vi "Refprop_Example_main_V10.vi"() -> ()   [LabVIEW 2016]
doc: "Sample vi to demonstrate the use of REFPROP in LabVIEW developed by Ken Pop Yan Ding.\nThare are also some VIs written by Greg Sussman in this example.Thanks Greg Sussman."
panel:
  out "INFO_OUT":T1
  out "1st run":bool
  out "name out":string
  out "o2":string
  out "o1":string
  out "error out":errorcluster caption="Error Out"
  out "refprop _main_directory":string
  out "DLL Version Number":dbl format="%.2g"
  in  "InpCode":T2(ring)=enum."TP"
  out "data":string[][](table)=[["0", "T", "40.917420"], ["1", "P", "632.917420"], ["2", "H", "466.332574"], ["3", "S", "2.054657"], ["4", "DV", "18.926081"], ["5", "DL", "18.926081"], ["6", "E", "432.891028"], ["7", "CV", "0.758226"], ["8", "CP", "0.924261"], ["9", "W", "194.299169"], ["10", "Q", "998.000000"]]
  in  "input_2":dbl=632.0
  in  "input_1":dbl=40.0
  in  "Units":enum16{"SI"}(ring)
  in  "Fluid Name":u16(ring)=17 items=["R401A.MIX", "R401B.MIX", "R401C.MIX", "R402A.MIX", "R402B.MIX", "R403A.MIX", "R403B.MIX", "R405A.MIX", "R406A.MIX", "R407A.MIX", "R407B.MIX", "R407C.MIX", "R407D.MIX", "R407E.MIX", "R408A.MIX", "R409A.MIX", "R409B.MIX", "R410A.MIX", "R410B.MIX", "R411A.MIX", "R411B.MIX", "R412A.MIX", "R413A.MIX", "R414B.MIX", "R500.MIX", "R501.MIX", "R502.MIX", "R503.MIX", "R504.MIX", "R507A.MIX", "R508A.MIX", "R508B.MIX", "R509A.MIX", "ammonia.fld", "butane.fld", "ethane.fld", "propane.fld", "R11.fld", "R113.fld", "R114.fld", "R115.fld", "R116.fld", "R12.fld", "R123.fld", "R124.fld", "R125.fld", "R13.fld", "R134a.fld", "R141b.fld", "R142b.fld", "R143a.fld", "R152a.fld", "R218.fld", "R22.fld", "R227ea.fld", "R23.fld", "R236ea.fld", "R236fa.fld", "R245ca.fld", "R245fa.fld", "R32.fld", "R41.fld", "RC318.fld", "water.fld"]
  # "-->"
  # "-->"
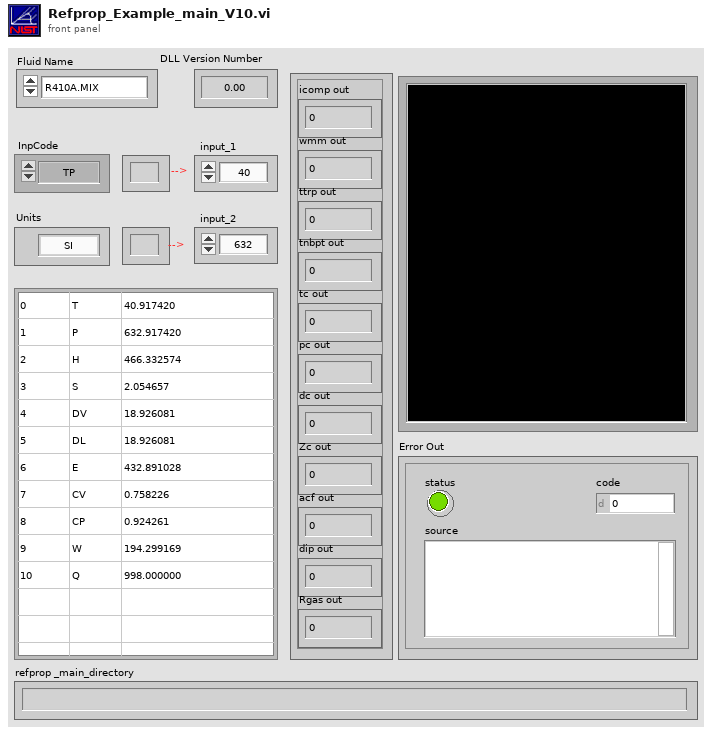
[diagram p1: front panel]
types:
  T1 = cluster{"icomp out":i32, "wmm out":dbl, "ttrp out":dbl, "tnbpt out":dbl, "tc out":dbl, "pc out":dbl, "dc out":dbl, "Zc out":dbl, "acf out":dbl, "dip out":dbl, "Rgas out":dbl}
  T2 = enum16{"0", "PS", "HS", "T", "P", "TP", "TH", "TS", "PH", "PQ", "TQ"}
  T3 = typedef "Mixture Composition cluster_d.ctl" = cluster{"Mixture Name":string, "Molecular weight (g/mol)":dbl, "Critical temperature (K)":dbl, "Critical Pressure (kPa)":dbl, "Critical Density (mol/L)":dbl, "# Components":i32, "Fluid File Paths":path[], "Component molar fractions":dbl[], "Refprop Main Directory":path, "DLL Version Number":dbl}
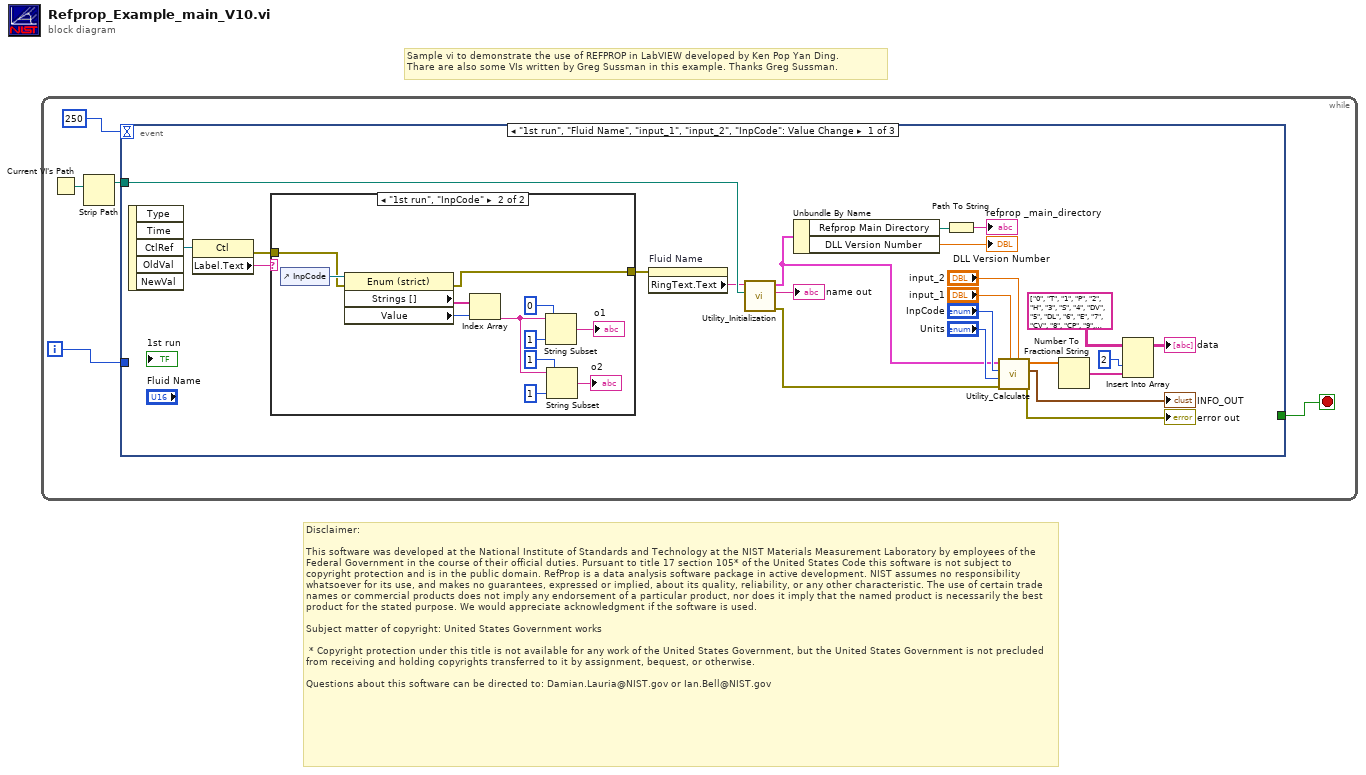
[diagram p0: block diagram]
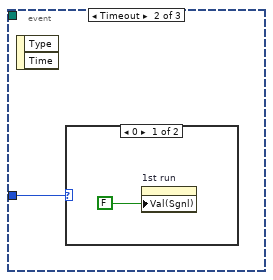
[diagram p3: hidden frame]
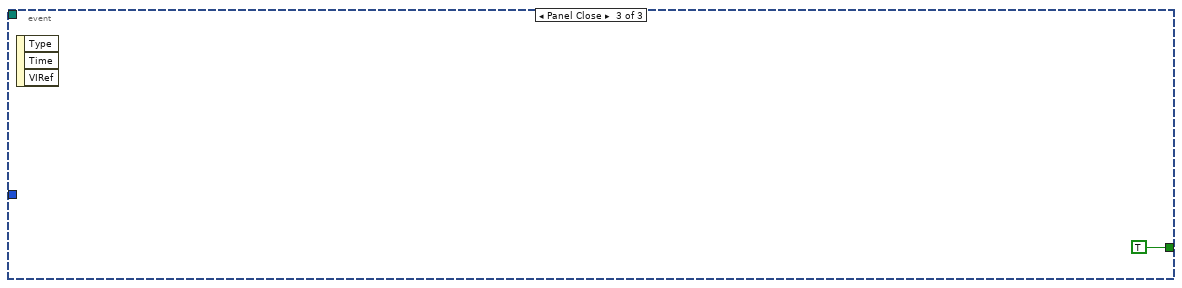
[diagram p5: hidden frame]
diagram:
  # "Sample vi to demonstrate the use of REFPROP in LabVIEW developed by Ken Pop Yan Ding.\nThare are also some VIs written by Greg Sussman in this example. Thanks Greg Sussman."
  # "Disclaimer:\n\nThis software was developed at the National Institute of Standards and Technology at the NIST Materials Measurement Laboratory by employees of the Federal Government in the course of their official duties. Pursuant to title 17 section 105* of the United States Code this software is not subject to copyright protection and is in the public domain. RefProp is a data analysis software package in active development. NIST assumes no responsibility whatsoever for its use, and makes no guarantees, expressed or implied, about its quality, reliability, or any other characteristic. The use of certain trade names or commercial products does not imply any endorsement of a particular product, nor does it imply that the named product is necessarily the best product for the stated purpose. We would appreciate acknowledgment if the software is used.\n \nSubject matter of copyright: United States Government works\n  \n * Copyright protection under this title is not available for any work of the United States Government, but the United States Government is not precluded from receiving and holding copyrights transferred to it by assignment, bequest, or otherwise.\n\nQuestions about this software can be directed to: Damian.Lauria@NIST.gov or Ian.Bell@NIST.gov"
  n1 = while {
    i -> [w3]
    stop <- w5 stop-if-true
    n2 = Current VI's Path() -> (path=w2:path)
    n3 = Strip Path(path=w2) -> (stripped path=w1:path)  [unwired: 1 out]
    n4 = event shown="[0] \"1st run\", \"Fluid Name\", \"input_1\", \"input_2\", \"InpCode\": Value Change" {
      selector: _ -> [_ _ _]
      dyn-events: _ -> [_ _ _]
      timeout: 250 -> [_ _ _]
      tunnel: w1 -> [w28 _ _]
      tunnel: [_ _ TRUE] -> w5
      tunnel: w3 -> [_ w42 _]
      event "1st run", "Fluid Name", "input_1", "input_2", "InpCode": Value Change {
        n5 = event-data() -> ("CtlRef"=w27:refnum<vi>)  [unwired: 1 in, 4 out]
        n6 = property class="Ctl"(reference=w27) -> (error out=w9:errorcluster, "Label.Text"=w26:string)  [unwired: 1 in, 1 out]
        n7 = case shown="\"1st run\", \"InpCode\"" w26 {
          tunnel: w9 -> [w29 w31]
          tunnel: [w29 w30] -> w8
          frame "假", Default {
          }
          frame "1st run", "InpCode" {
            n8 = control-ref of="InpCode"() -> (w32:refnum<vi>)
            n9 = property class="Enum (strict)"(reference=w32, error in=w31) -> (error out=w30:errorcluster, "Strings []"=w41:string[], "Value"=w40:T2)  [unwired: 1 out]
            n10 = Index Array(array=w41, index=w40) -> (element=w37:string)
            n11 = String Subset(string=w37, offset (0)=0 ("偏移量(0)"), length (rest)=1 ("长度（剩余）")) -> (substring=→"o1":string)
            n12 = String Subset(string=w37, offset (0)=1 ("偏移量(0)"), length (rest)=1 ("长度（剩余）")) -> (substring=→"o2":string)
          }
        }
        n13 = property on="Fluid Name" class="Ring (strict)"(error in=w8) -> ("RingText.Text"=w21:string)  [unwired: 1 in, 2 out]
        n14 = call "Utility_Initialization.vi"("path"=w28, "Fluidofinterest"=w21) -> ("error out"=w14:errorcluster, "name out"=→"name out":string, "Mixure Cluster out"=w7:T3)  [unwired: 7 in]
        n15 = Unbundle By Name(w7) -> ("Refprop Main Directory"=w11:path, "DLL Version Number"=→"DLL Version Number":dbl)
        n16 = Path To String(path=w11) -> (string=→"refprop _main_directory":string)
        n17 = call "Utility_Calculate.vi"("input_2"="input_2", "input_1"="input_1", "error in"=w14, "units"="Units", "InpCode"="InpCode", "Mixure Cluster"=w7) -> ("error out"=→"error out":errorcluster, "INFO_OUT"=→"INFO_OUT":T1, "dataout"=w17:dbl[])  [unwired: 3 in]
        n18 = Number To Fractional String(number=w17) -> (F-format string=w24:string[])  [unwired: 3 in]
        n19 = Insert Into Array(array=string[][] [["0", "T"], ["1", "P"], ["2", "H"], ["3", "S"], ["4", "DV"], ["5", "DL"], ["6", "E"], ["7", "CV"], ["8", "CP"], ["9", "W"], ["10", "Q"]] ("数组"), index (col)=2 ("禁用的索引 (列)"), new element=w24) -> (→"data":string[][])  [unwired: 1 in]
      }
      event Timeout {
        n20 = event-data() -> ()  [unwired: 1 in, 2 out]
        n21 = case shown="0" w42 {
          frame 0 {
            n22 = property on="1st run" class="Bool (strict)"("Val(Sgnl)"=FALSE ("值(信号)")) -> ()  [unwired: 2 in, 2 out]
          }
          frame 1, Default {
          }
        }
      }
      event Panel Close {
        n23 = event-data() -> ()  [unwired: 1 in, 3 out]
      }
    }
  }
